vi "SP Handle Autoscaling.vi"(8 "error in (no error)":errorcluster, 9 "Channel":i8=1 min=1 max=99 step=1, 10 "CH Control":T1={"Trace On"=TRUE, "Measure"=0, "Format"=0, "Autoscale"=TRUE, "Reference"=0.0, "\nRefUnit"="dB/Div", "Position"=5.0, "Scale"=10.0, "ScaleUnit"="dB/Div", "LimitOn"=TRUE, "LimitFill"=FALSE, "Display Data"=0, "Show Markers"=TRUE, "SXX"=""} {"Reference" format="%#.2g"; "Display Data" items=["Data", "Memory", "Data/Memory"]; "Format" items=["Log Mag", "Phase", "Expanded Phase", "Delay", "Smith", "Polar", "Lin Mag", "SWR", "Loss", "Real", "Imaginary"]; "Scale" min=0.001 step=1.0 format="%#.2g"; "Position" min=0.0 max=10.0}, 11 "Plot Reference":refnum<vi>) -> (0 "error out":errorcluster, 2 "new CH Control":T1={"Trace On"=TRUE, "Measure"=0, "Format"=0, "Autoscale"=TRUE, "Reference"=0.0, "\nRefUnit"="dB/Div", "Position"=5.0, "Scale"=10.0, "ScaleUnit"="dB/Div", "LimitOn"=TRUE, "LimitFill"=FALSE, "Display Data"=0, "Show Markers"=TRUE, "SXX"=""} {"Reference" format="%#.2g"; "Display Data" items=["Data", "Memory", "Data/Memory"]; "Format" items=["Log Mag", "Phase", "Expanded Phase", "Delay", "Smith", "Polar", "Lin Mag", "SWR", "Loss", "Real", "Imaginary"]; "Scale" min=0.001 step=1.0 format="%#.2g"; "Position" min=0.0 max=10.0}, 3 "Plot Reference":refnum<vi>)   [LabVIEW 2011]
uses:
  TypeDefs/SP Display Trace Controls.ctl
  TypeDefs/SP Display Format.ctl
  TypeDefs/SP Display Data.ctl
  TypeDefs/SP Plot Cluster Object.ctl
panel:
  # "Div"
  # "Div"
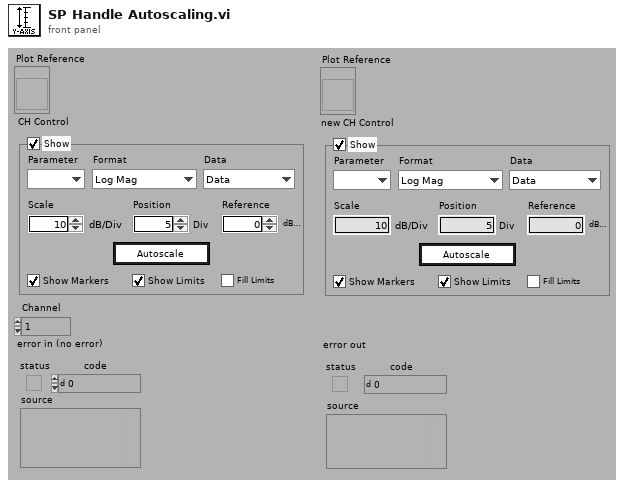
[diagram p1: front panel]
types:
  T1 = typedef "SP Display Trace Controls.ctl" = cluster{"Trace On":bool, "Measure":i32, "Format":T2, "Autoscale":bool, "Reference":dbl, "\nRefUnit":string, "Position":dbl, "Scale":dbl, "ScaleUnit":string, "LimitOn":bool, "LimitFill":bool, "Display Data":T3, "Show Markers":bool, "SXX":string}
  T2 = typedef "SP Display Format.ctl" = i32
  T3 = typedef "SP Display Data.ctl" = u16
  T4 = typedef "SP Plot Cluster Object.ctl" = enum16{"Plot", "CH Reference", "CH Label", "Start Label", "Stop Label", "Units Label", "Selected?", "CH Markers"}
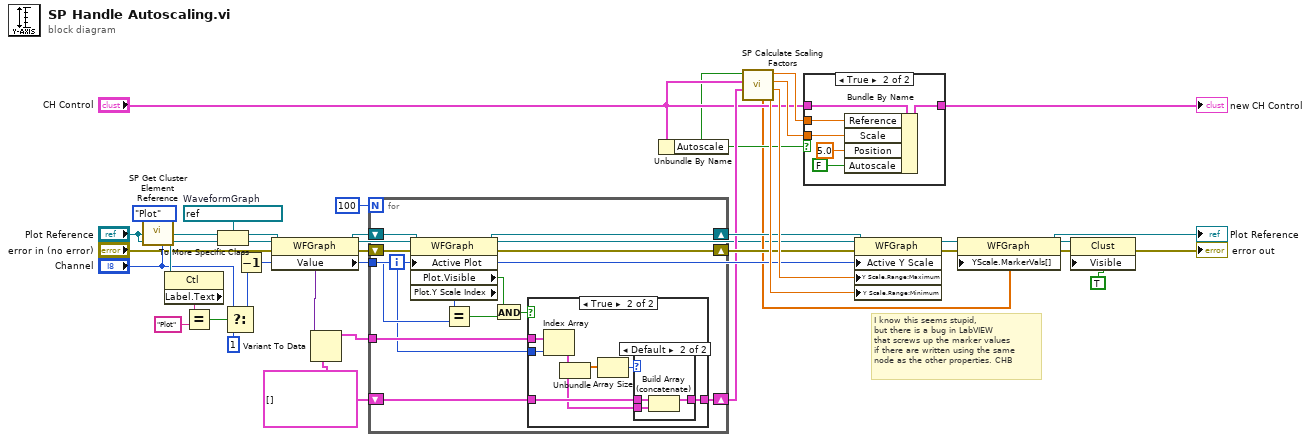
[diagram p0: block diagram]
diagram:
  w13 = cluster{"X":dbl[], "Y":dbl[]}[] [] ("X-Y Plot")
  w33 = refnum<vi> refnum  # WaveformGraph
  # "I know this seems stupid,\nbut there is a bug in LabVIEW\nthat screws up the marker values\nif there are written using the same\nnode as the other properties. CHB"
  n1 = call "SP Get Cluster Element Reference.vi"("Channel"="Channel", "Element"=SP_Plot_Cluster_Object."Plot", "Plot Reference"="Plot Reference") -> ("Element Reference"=w30:refnum<vi>)  [unwired: 6 out]
  n2 = property class="Ctl"(reference=w30) -> ("Label.Text"=w32:string)  [unwired: 1 in, 2 out]
  n3 = Equal?(x=w32, y="Plot") -> (x = y?=w26:bool)
  n4 = To More Specific Class(target class=w33, reference=w30) -> (specific class reference=w18:refnum<vi>)  [unwired: 1 in, 1 out]
  n5 = Select(t="Channel", s=w26, f=i8 1 ("Channel")) -> (s? t:f=w28:i8)
  n6 = Decrement(x=w28) -> (x-1=w20:i8)
  n7 = property on="Property Node" class="WFGraph"(reference=w18, error in="error in (no error)") -> (reference out=w17:refnum<vi>, error out=w16:errorcluster, "Value"=w15:variant)
  n8 = Variant To Data(type=w13, Variant=w15) -> (data=w14:cluster{"X":dbl[], "Y":dbl[]}[])  [unwired: 1 in, 1 out]
  n9 = for {
    N: 100 -> [_]
    shift-right: [w46] -> w22
    shift-left: w16 -> [w48]
    shift-right: [w47] -> w23
    shift-left: w17 -> [w49]
    tunnel: w20 -> [w45]
    tunnel: w14 -> [w40]
    shift-right: [w37] -> w12
    shift-left: w13 -> [w38]
    i -> [w39]
    n10 = property on="Property Node" class="WFGraph"(reference=w49, error in=w48, "Active Plot"=w39) -> (reference out=w47:refnum<vi>, error out=w46:errorcluster, "Plot.Visible"=w43:bool, "Plot.Y Scale Index"=w44:u32)
    n11 = Equal?(x=w44, y=w45) -> (x = y?=w42:bool)
    n12 = And(x=w43, y=w42) -> (x .and. y?=w41:bool)
    n13 = case shown="True" w41 {
      tunnel: w40 -> [_ w57]
      tunnel: w39 -> [_ w56]
      tunnel: w38 -> [w50 w55]
      tunnel: [w50 w54] -> w37
      frame False {
      }
      frame True {
        n14 = Index Array(array=w57, index=w56) -> (element=w53:cluster{"X":dbl[], "Y":dbl[]})
        n15 = Unbundle(w53) -> ("X"=w52:dbl[])  [unwired: 1 out]
        n16 = Array Size(array=w52) -> (size(s)=w51:i32)
        n17 = case shown="Default" w51 {
          tunnel: w55 -> [w58 w61]
          tunnel: [w58 w60] -> w54
          tunnel: w53 -> [_ w59]
          frame 0 {
          }
          frame Default {
            n18 = Build Array (concatenate)(w61, w59) -> (w60:cluster{"X":dbl[], "Y":dbl[]}[])
          }
        }
      }
    }
  }
  n19 = Unbundle By Name("CH Control") -> ("Autoscale"=w9:bool)
  n20 = call "SP Calculate Scaling Factors.vi"("X-Y Plot"=w12, "CH Control"="CH Control", "Autoscale?"=w9) -> ("Y Min"=w24:dbl, "Y Max"=w25:dbl, "Scale"=w35:dbl, "Reference"=w34:dbl, "Y Markers"=w5:dbl[])  [unwired: 4 out]
  n21 = case shown="True" w9 {
    tunnel: [w62 w68] -> w36
    tunnel: w35 -> [_ w67]
    tunnel: w34 -> [_ w65]
    tunnel: "CH Control" -> [w62 w64]
    frame False {
    }
    frame True {
      n22 = Bundle By Name(cluster=w64, "Reference"=w65, "Scale"=w67, "Position"=5.0, "Autoscale"=FALSE) -> (w68:T1)
    }
  }
  "new CH Control" <- w36
  n23 = property on="Property Node" class="WFGraph"(reference=w23, error in=w22, "Active Y Scale"=w20, "Y Scale.Range:Maximum"=w25, "Y Scale.Range:Minimum"=w24) -> (reference out=w6:refnum<vi>, error out=w7:errorcluster)
  n24 = property on="Property Node" class="WFGraph"(reference=w6, error in=w7, "YScale.MarkerVals[]"=w5) -> (reference out=→"Plot Reference":refnum<vi>, error out=w3:errorcluster)
  n25 = property on="Property Node" class="Clust"(reference="Plot Reference", error in=w3, "Visible"=TRUE) -> (error out=→"error out":errorcluster)  [unwired: 1 out]
